vi "Grap Image with trigger test.vi"(0 "Refnum in":T3, 1 "Process Queueu":refnum<queue>, 2 "Live Queue":refnum<queue>, 3 "Status Queueu":refnum<queue>, 4 "Trigger is on ?":bool=TRUE, 5 "error in":errorcluster) -> (14 "Refnum out":T3, 16 "Pass?":bool, 19 "error out":errorcluster)   [LabVIEW 2015]
uses:
  <vilib>/userdefined/High Color/IMAQdx.ctl
  <vilib>/vision/driver/NI_Vision_Acquisition_Software.lvlib
panel:
  in  "Exit":bool
  out "Process Image":T1(plugin-control)
  out "Execution:State":T2(ring)
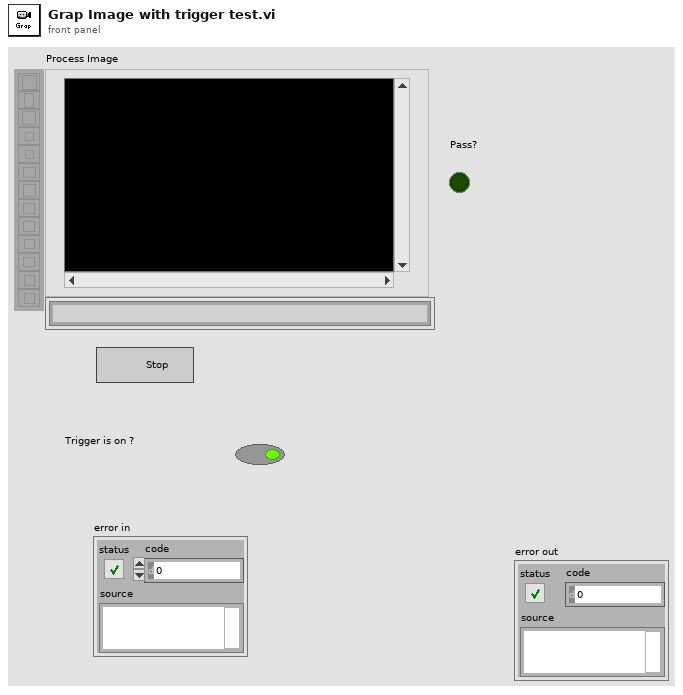
[diagram p1: front panel]
types:
  T1 = typedef "IMAQ Image.ctl" = refnum<image>
  T2 = enum32{"Bad", "Idle", "Run top level", "Running"}
  T3 = typedef "IMAQdx.ctl" = refnum<k21>
  T4 = cluster{"Message":string, "Message Data":variant}
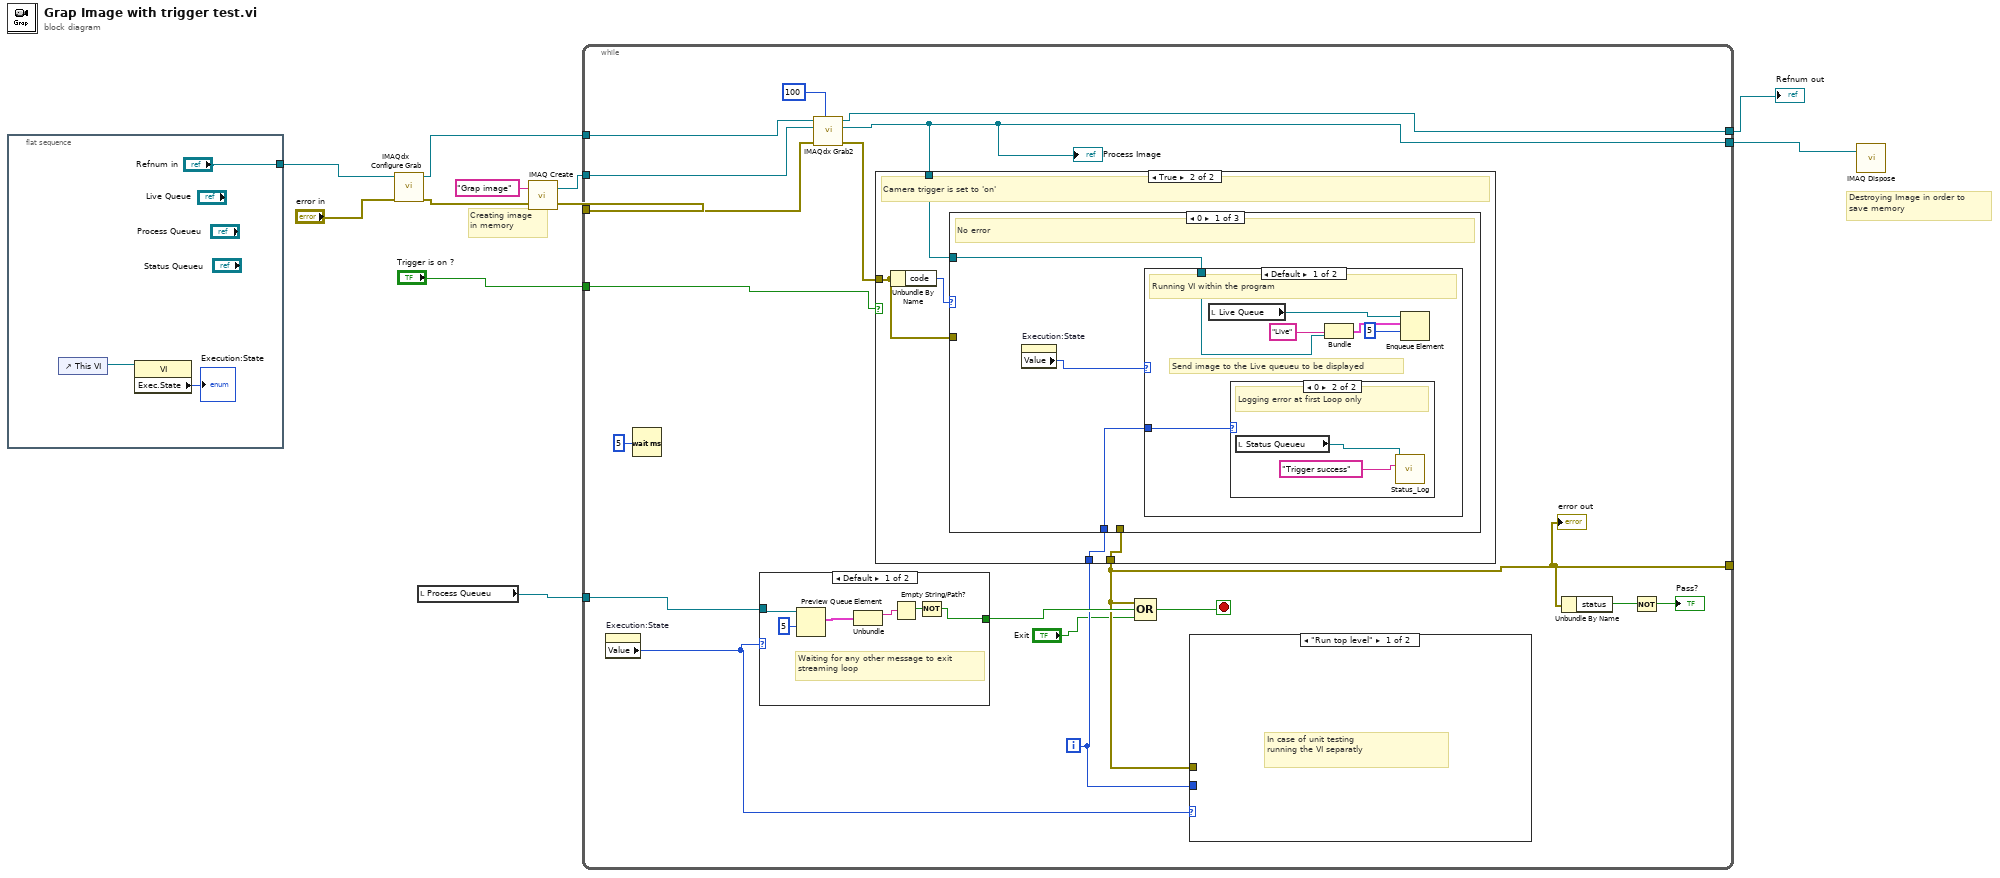
[diagram p0: block diagram]
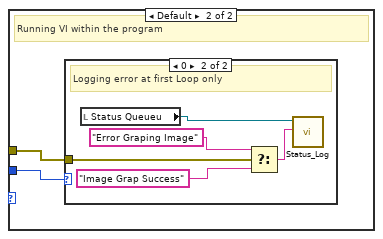
[diagram p2: hidden frame]
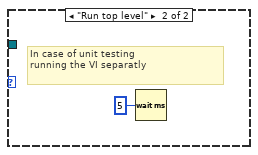
[diagram p4: hidden frame]
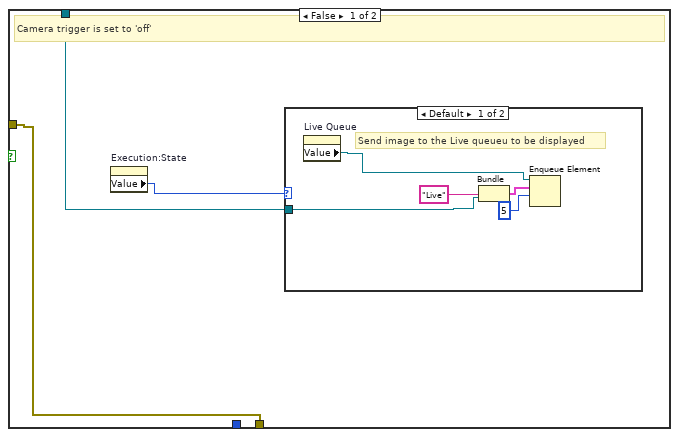
[diagram p5: hidden frame]
diagram:
  # "Destroying Image in order to\nsave memory"
  # "Creating image\nin memory"
  n1 = flat-sequence {
    tunnel: ["Refnum in"] -> w3
    frame #0 {
      n2 = control-ref of="This VI"() -> (w12:refnum<vi>)
      n3 = property class="VI"(reference=w12) -> ("Exec.State"=→"Execution:State":T2)  [unwired: 1 in, 2 out]
    }
  }
  n4 = call <vilib>:"IMAQdx Configure Grab.vi"("error in"="error in", "Session In"=w3) -> ("error out"=w10:errorcluster, "Session Out"=w6:T3)  [unwired: 8 in]
  n5 = local read "Process Queueu"() -> (w2:refnum<queue>)
  n6 = call "IMAQ Create"("Image Name"="Grap image", "error in (no error)"=w10) -> ("New Image"=w8:T1, "error out"=w11:errorcluster)  [unwired: 3 in]
  n7 = while {
    tunnel: w6 -> [w32]
    tunnel: w8 -> [w31]
    tunnel: [w20] -> w9
    tunnel: w11 -> [w30]
    tunnel: [w28] -> w5
    tunnel: [w17] -> _
    tunnel: w2 -> [w24]
    tunnel: "Trigger is on ?" -> [w23]
    i -> [w25]
    stop <- w29 stop-if-true
    n8 = property on="Execution:State" class="Enum (strict)"() -> ("Value"=w21:T2)  [unwired: 2 in, 2 out]
    n9 = Wait (ms)(milliseconds to wait=u32 5) -> ()  [unwired: 1 out]
    n10 = case shown="Default" w21 {
      tunnel: [w41 _] -> w26
      tunnel: w24 -> [w40 _]
      frame Default {
        # "Waiting for any other message to exit\nstreaming loop"
        n11 = Preview Queue Element(queue=w40, timeout in ms (-1)=5) -> (element=w45:T4)  [unwired: 1 in, 3 out]
        n12 = Unbundle(w45) -> ("Message"=w43:string)  [unwired: 1 out]
        n13 = Empty String/Path?(string/path=w43) -> (empty?=w42:bool)
        n14 = Not(x=w42) -> (.not. x?=w41:bool)
      }
      frame "Run top level" {
        # "In case of unit testing\nrunning the VI separatly"
        n15 = Wait (ms)(milliseconds to wait=u32 5) -> ()  [unwired: 1 out]
      }
    }
    n16 = call <vilib>:"IMAQdx Grab2.vi"("Timeout (ms)"=100, "error in"=w30, "Image In"=w31, "Session In"=w32) -> ("error out"=w22:errorcluster, "Image Out"=w20:T1, "Session Out"=w28:T3)  [unwired: 4 in, 1 out]
    "Process Image" <- w20
    n17 = case shown="True" w23 {
      tunnel: w20 -> [w49 w58]
      tunnel: w22 -> [w47 w56]
      tunnel: [w47 w55] -> w17
      tunnel: w25 -> [_ w57]
      frame False {
        # "Camera trigger is set to 'off'"
        n18 = property on="Execution:State" class="Enum (strict)"() -> ("Value"=w48:T2)  [unwired: 2 in, 2 out]
        n19 = case shown="Default" w48 {
          tunnel: w49 -> [w54 _]
          frame Default {
            # "Send image to the Live queueu to be displayed"
            n20 = property on="Live Queue" class="TypRef (strict)"() -> ("Value"=w51:refnum<queue>)  [unwired: 2 in, 2 out]
            n21 = Bundle("Live", "Image Out"=w54) -> (w53:cluster{string, "Image Out":T1})  [unwired: 1 in]
            n22 = Enqueue Element(queue=w51, element=w53, timeout in ms (-1)=5) -> ()  [unwired: 1 in, 3 out]
          }
          frame "Run top level" {
            # "In case of unit testing\nrunning the VI separatly in test stand"
          }
        }
      }
      frame True {
        # "Camera trigger is set to 'on'"
        n23 = Unbundle By Name(w56) -> ("code"=w59:i32)
        n24 = case shown="0" w59 {
          tunnel: w58 -> [w62 _ _]
          tunnel: w57 -> [w61 _ _]
          tunnel: w56 -> [_ w71 _]
          tunnel: [_ w71 _] -> w55
          frame 0 {
            # "No error"
            n25 = property on="Execution:State" class="Enum (strict)"() -> ("Value"=w60:T2)  [unwired: 2 in, 2 out]
            n26 = case shown="Default" w60 {
              tunnel: w62 -> [w66 _]
              tunnel: w61 -> [w65 _]
              frame Default {
                # "Send image to the Live queueu to be displayed"
                # "Running VI within the program"
                n27 = local read "Live Queue"() -> (w64:refnum<queue>)
                n28 = case shown="0" w65 {
                  frame Default {
                  }
                  frame 0 {
                    # "Logging error at first Loop only"
                    n29 = local read "Status Queueu"() -> (w69:refnum<queue>)
                    n30 = call "Status_Log.vi"("String"="Trigger success", "Status Queue"=w69) -> ()  [unwired: 9 in, 1 out]
                  }
                }
                n31 = Bundle("Live", "Image Out"=w66) -> (w68:cluster{string, "Image Out":T1})  [unwired: 1 in]
                n32 = Enqueue Element(queue=w64, element=w68, timeout in ms (-1)=5) -> ()  [unwired: 1 in, 3 out]
              }
              frame "Run top level" {
                # "In case of unit testing\nrunning the VI separatly"
              }
            }
          }
          frame Default {
            # "Any other error in graping"
          }
          frame -1074360293 {
            # "Time out error\nhas to be ignored \nto wait for trigger"
          }
        }
      }
    }
    "error out" <- w17
    n33 = Compound Arithmetic op=OR(w17, w26, "Exit") -> (w29:bool)
    n34 = case shown="\"Run top level\"" w21 {
      tunnel: w25 -> [_ w34]
      tunnel: w17 -> [_ w33]
      frame "Run top level" {
        # "In case of unit testing\nrunning the VI separatly"
      }
      frame Default {
        # "Running VI within the program"
        n35 = case shown="0" w34 {
          tunnel: w33 -> [_ w39]
          frame Default {
          }
          frame 0 {
            # "Logging error at first Loop only"
            n36 = local read "Status Queueu"() -> (w35:refnum<queue>)
            n37 = Select(t="Error Graping Image", s=w39, f="Image Grap Success") -> (s? t:f=w36:string)
            n38 = call "Status_Log.vi"("String"=w36, "Status Queue"=w35) -> ()  [unwired: 9 in, 1 out]
          }
        }
      }
    }
    n39 = Unbundle By Name(w17) -> ("status"=w18:bool)
    n40 = Not(x=w18) -> (.not. x?=→"Pass?":bool)
  }
  "Refnum out" <- w5
  n41 = call "IMAQ Dispose"("Image"=w9) -> ()  [unwired: 5 in, 1 out]
